vi "Get Chars.vi"(7 "Width":i32, 8 "error in (no error)":errorcluster, 11 "TermLine in":refnum<class "TermLine.lvclass">) -> (0 "error out":errorcluster, 2 "TermChars":T1[](array[typedef]), 3 "TermLine out":refnum<class "TermLine.lvclass">)   [LabVIEW 2020, in "Terminal.lvlib" / "TermLine.lvclass"]
uses:
  TermLine.lvclass
  TermLine.lvclass/TermLine.ctl
  Term Char.ctl
  Terminal.lvlib
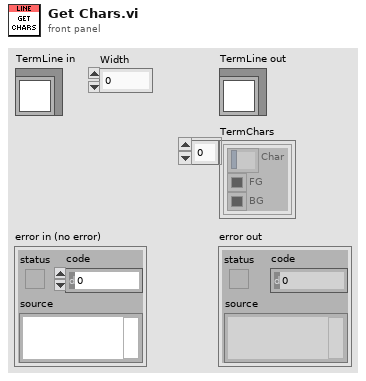
[diagram p1: front panel]
types:
  T1 = typedef "Terminal.lvlib/Term Char.ctl" = cluster{"Char":string, "FG":u32, "BG":u32}
  T2 = typedef "Terminal.lvlib/TermLine.lvclass/Ref Data.ctl" = cluster{"Chars":T1[], "Width":i32}
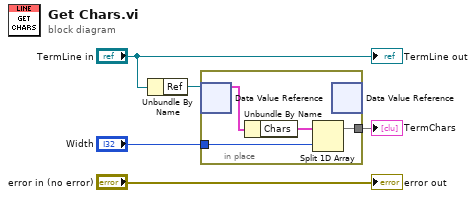
[diagram p0: block diagram]
diagram:
  n1 = Unbundle By Name("TermLine in") -> ("Ref"=w4:refnum<data-value>)
  n2 = in-place {
    in-place-border: "Width" -> [w7]
    in-place-border: [w6] -> w1
    n3 = in-place-dvr #1(w4) -> (w9:T2)  [unwired: 1 out]
    n4 = Unbundle By Name(w9) -> ("Chars"=w8:T1[])
    n5 = Split 1D Array(array=w8, index=w7) -> (first subarray=w6:T1[])  [unwired: 1 out]
    n6 = in-place-dvr #1() -> ()  [unwired: 1 in, 2 out]
  }
  "TermChars" <- w1
  "error out" <- "error in (no error)"
  "TermLine out" <- "TermLine in"
